vi "Create Parameter Group.vi"(8 "error in (no error)":errorcluster, 9 "Control Properties":T1(array[cluster]), 10 "Group name":string, 11 "CD Parameter Manager in":refnum<class "CD Parameter Manager.lvclass">) -> (0 "error out":errorcluster, 3 "CD Parameter Manager out":refnum<class "CD Parameter Manager.lvclass">)   [LabVIEW 2019, in "CD Parameter Manager API.lvlib" / "CD Parameter Manager.lvclass"]
uses:
  CD Parameter Manager.lvclass
  Parameter Class/Parameter.lvclass
  CD Parameter Manager.lvclass/CD Parameter Manager.ctl
  Double Parameter Class/Double Parameter.lvclass
  C:/Repositories/CSD_Custom_Device/CSD_Custom_Device/Source/Libraries/CD Parameter Manager API/Parameter Class/Parameter.lvclass
  I32 Parameter Class/I32 Parameter.lvclass
  String Parameter Class/String Parameter.lvclass
  Boolean Parameter Class/Boolean Parameter.lvclass
  File Path Parameter Class/File Path Parameter.lvclass
  Parameter Class/Parameter.lvclass/Parameter.ctl
  Parameter Class/Member Accessors/Write Control label.vi
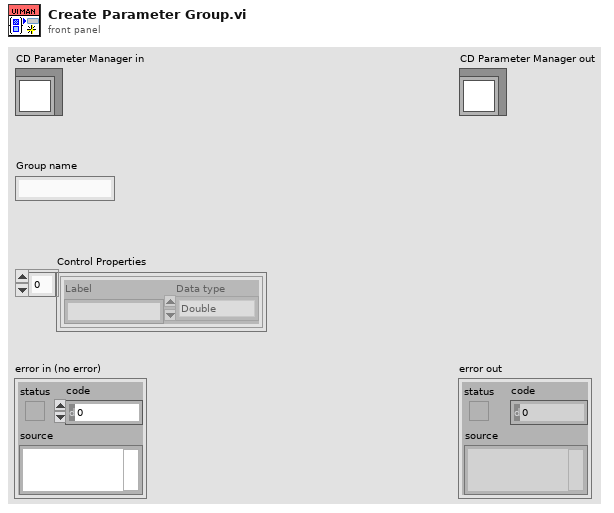
[diagram p1: front panel]
types:
  T1 = cluster{"Label":string, "Data type":enum16{"Double", "I32", "Boolean", "String", "File Path"}}[]
  T2 = cluster{"Group name":string, "Controls":refnum<class "Parameter.lvclass">[]}
  T3 = enum16{"Double", "I32", "Boolean", "String", "File Path"}
  T4 = cluster{"Group name":string, "Controls":refnum<class "Parameter.lvclass">[]}[]
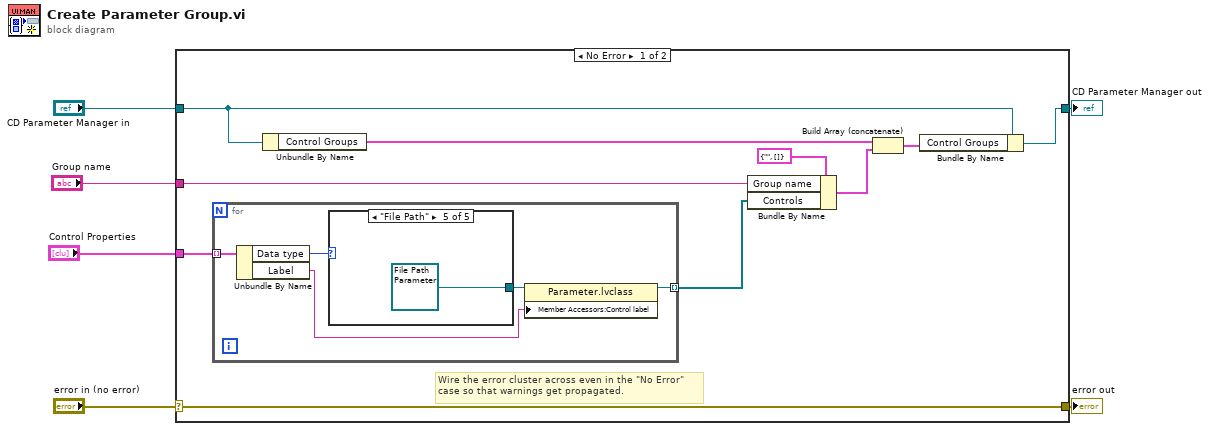
[diagram p0: block diagram]
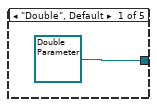
[diagram p2: hidden frame]
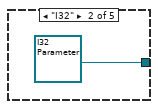
[diagram p3: hidden frame]
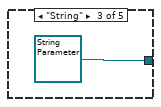
[diagram p4: hidden frame]
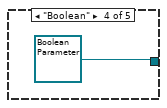
[diagram p5: hidden frame]
diagram:
  n1 = case shown="No Error" "error in (no error)" {
    selector: "error in (no error)" -> [w16 w28]
    tunnel: [w16 w28] -> w5
    tunnel: [w15 w27] -> w3
    tunnel: "CD Parameter Manager in" -> [w14 w27]
    tunnel: "Control Properties" -> [w11 _]
    tunnel: "Group name" -> [w9 _]
    frame No Error {
      # "Wire the error cluster across even in the \"No Error\"\ncase so that warnings get propagated."
      n2 = for {
        tunnel: w11 -> [w21] mode=indexing
        tunnel: [w18] -> w8 mode=indexing
        n3 = Unbundle By Name(w21) -> ("Data type"=w20:T3, "Label"=w17:string)
        n4 = case shown="\"File Path\"" w20 {
          tunnel: [refnum<class "Double Parameter.lvclass"> refnum ("CD Parameter Manager API.lvlib:Double Parameter.lvclass") refnum<class "I32 Parameter.lvclass"> refnum ("CD Parameter Manager API.lvlib:I32 Parameter.lvclass") refnum<class "String Parameter.lvclass"> refnum ("CD Parameter Manager API.lvlib:String Parameter.lvclass") refnum<class "Boolean Parameter.lvclass"> refnum ("CD Parameter Manager API.lvlib:Boolean Parameter.lvclass") refnum<class "File Path Parameter.lvclass"> refnum ("CD Parameter Manager API.lvlib:File Path Parameter.lvclass")] -> w19
          frame "Double", Default {
          }
          frame "I32" {
          }
          frame "String" {
          }
          frame "Boolean" {
          }
          frame "File Path" {
          }
        }
        n5 = property class="Parameter.lvclass"(reference=w19, "Member Accessors:Control label"=w17) -> (reference out=w18:refnum<class "Parameter.lvclass">)  [unwired: 1 in, 1 out]
      }
      n6 = Unbundle By Name(w14) -> ("Control Groups"=w13:T4)
      n7 = Bundle By Name(cluster=T2 {"Group name"="", "Controls"=[]} ("Control Group"), "Group name"=w9, "Controls"=w8) -> (w7:T2)
      n8 = Build Array (concatenate)(w13, w7) -> (w12:T4)
      n9 = Bundle By Name(cluster=w14, "Control Groups"=w12) -> (w15:refnum<class "CD Parameter Manager.lvclass">)
    }
    frame Error {
    }
  }
  "error out" <- w5
  "CD Parameter Manager out" <- w3
